vi "Temperature Warnings.vi"() -> ()   [LabVIEW 2014]
doc: "在本练习中，将气象数据簇转换为自定义类型。"
uses:
  Weather Data.ctl
panel:
  out "气象数据输出":T1={"当前温度"=0.0, "最高温度"=0.0, "最低温度"=0.0, "温度警告？"=FALSE, "温度警告文本"="无警告", "单位"=0} {"单位" items=["摄氏", "华氏"]}
  in  "气象数据输入":T1={"当前温度"=0.0, "最高温度"=0.0, "最低温度"=0.0, "温度警告？"=FALSE, "温度警告文本"="无警告", "单位"=0} {"单位" items=["摄氏", "华氏"]}
  out "错误输出":cluster{"状态":bool, "代码":i32, "源":string}
  in  "错误输入":cluster{"状态":bool, "代码":i32, "源":string}
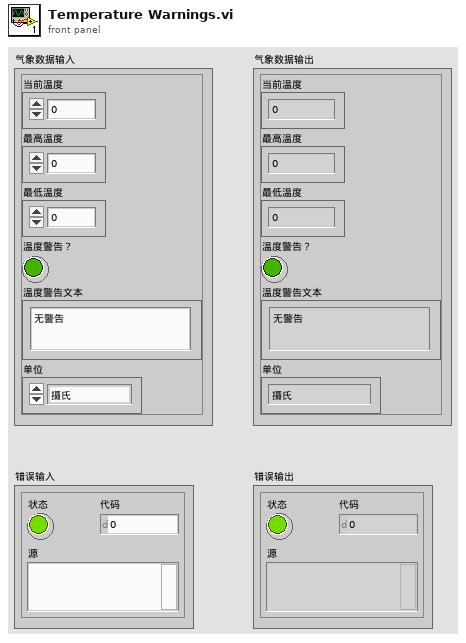
[diagram p1: front panel]
types:
  T1 = typedef "Weather Data.ctl" = cluster{"当前温度":dbl, "最高温度":dbl, "最低温度":dbl, "温度警告？":bool, "温度警告文本":string, "单位":u16}
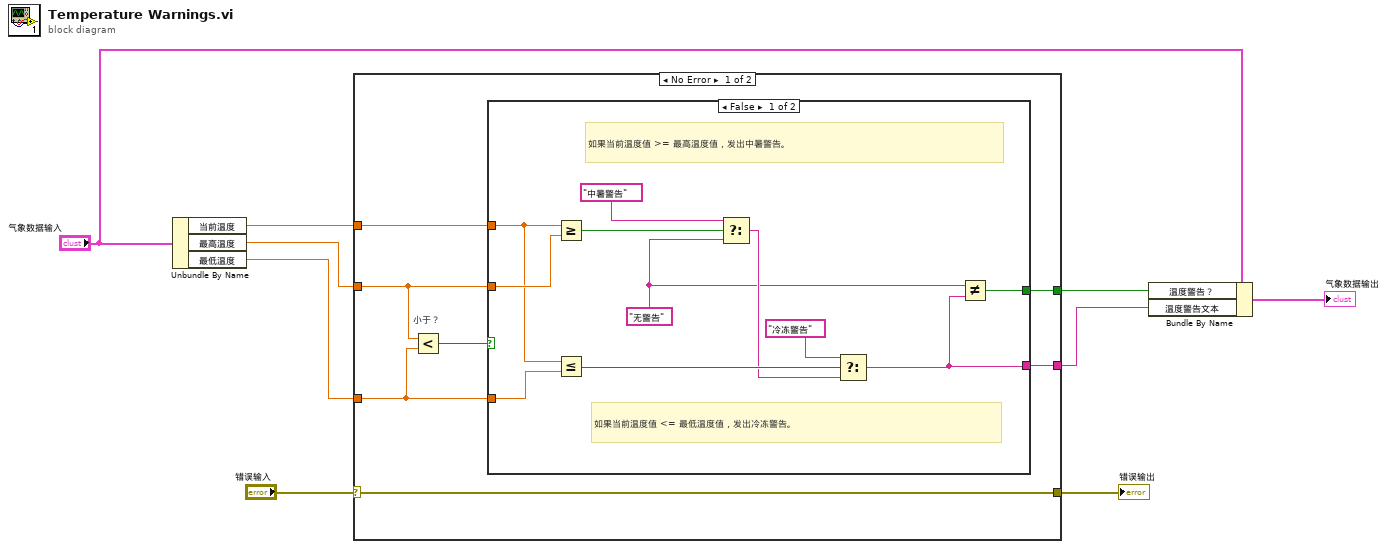
[diagram p0: block diagram]
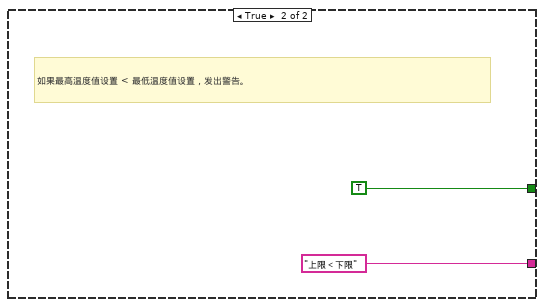
[diagram p2: hidden frame]
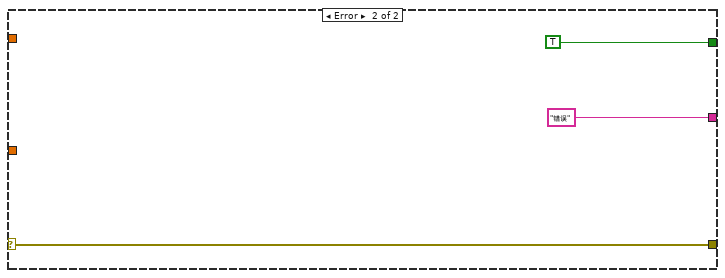
[diagram p3: hidden frame]
diagram:
  n1 = Unbundle By Name("气象数据输入") -> ("当前温度"=w3:dbl, "最高温度"=w5:dbl, "最低温度"=w4:dbl)
  n2 = case shown="No Error" "错误输入" {
    selector: "错误输入" -> [w14 w32]
    tunnel: [w16 "错误" ("f")] -> w1
    tunnel: [w15 TRUE] -> w2
    tunnel: [w14 w32] -> w6
    tunnel: w4 -> [w11 _]
    tunnel: w3 -> [w13 _]
    tunnel: w5 -> [w12 _]
    frame No Error {
      n3 = Less? "小于？"(x=w12, y=w11) -> (x < y?=w10:bool)
      n4 = case shown="False" w10 {
        tunnel: [w17 "上限＜下限" ("f")] -> w16
        tunnel: [w27 TRUE] -> w15
        tunnel: w12 -> [w26 _]
        tunnel: w11 -> [w23 _]
        tunnel: w13 -> [w19 _]
        frame False {
          w18 = "无警告" ("f")
          # "如果当前温度值 <= 最低温度值，发出冷冻警告。"
          # "如果当前温度值 >= 最高温度值，发出中暑警告。"
          n5 = Greater Or Equal?(x=w19, y=w26) -> (x >= y?=w25:bool)
          n6 = Less Or Equal?(x=w19, y=w23) -> (x <= y?=w21:bool)
          n7 = Select(t="中暑警告", s=w25, f=w18) -> (s? t:f=w20:string)
          n8 = Select(t="冷冻警告", s=w21, f=w20) -> (s? t:f=w17:string)
          n9 = Not Equal?(x=w18, y=w17) -> (x != y?=w27:bool)
        }
        frame True {
          # "如果最高温度值设置 < 最低温度值设置，发出警告。"
        }
      }
    }
    frame Error {
    }
  }
  "错误输出" <- w6
  n10 = Bundle By Name(cluster="气象数据输入", "温度警告？"=w2, "温度警告文本"=w1) -> (→"气象数据输出":T1)
